vi "Untitled 1.vi"() -> ()   [LabVIEW 2021]
uses:
  <vilib>/Analysis/NI_AALPro.lvlib
panel:
  out "x*y":dbl
  out "x/y":dbl
  out "unsigned 16bit integer":u32 format="%x"
  out "output variable":dbl
  in  "Freq":dbl
  out "XY Graph":cluster{dbl[], dbl[]}(graph)
  out "intercept":dbl
  out "slope":dbl
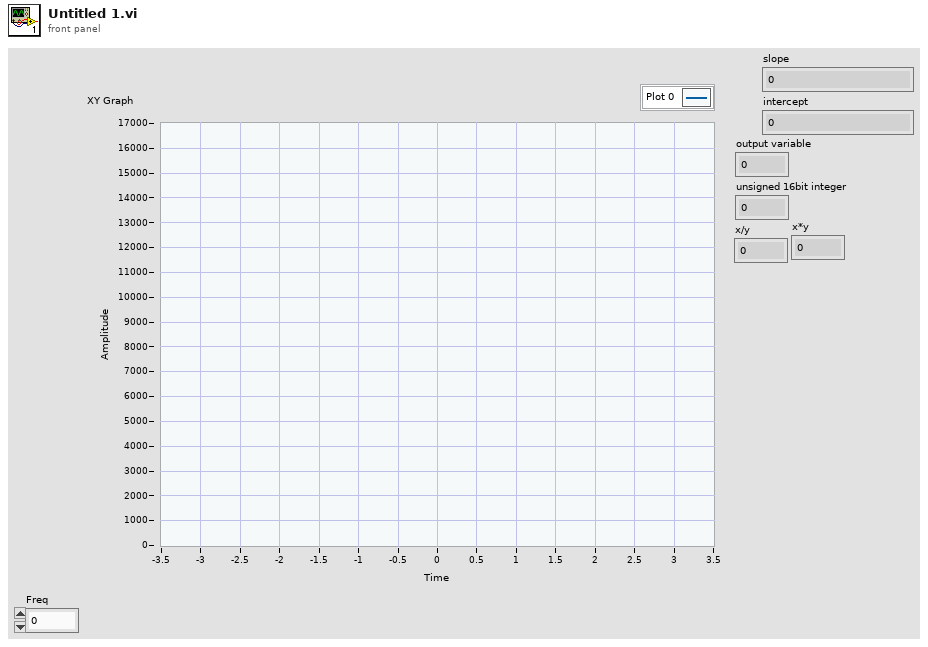
[diagram p1: front panel]
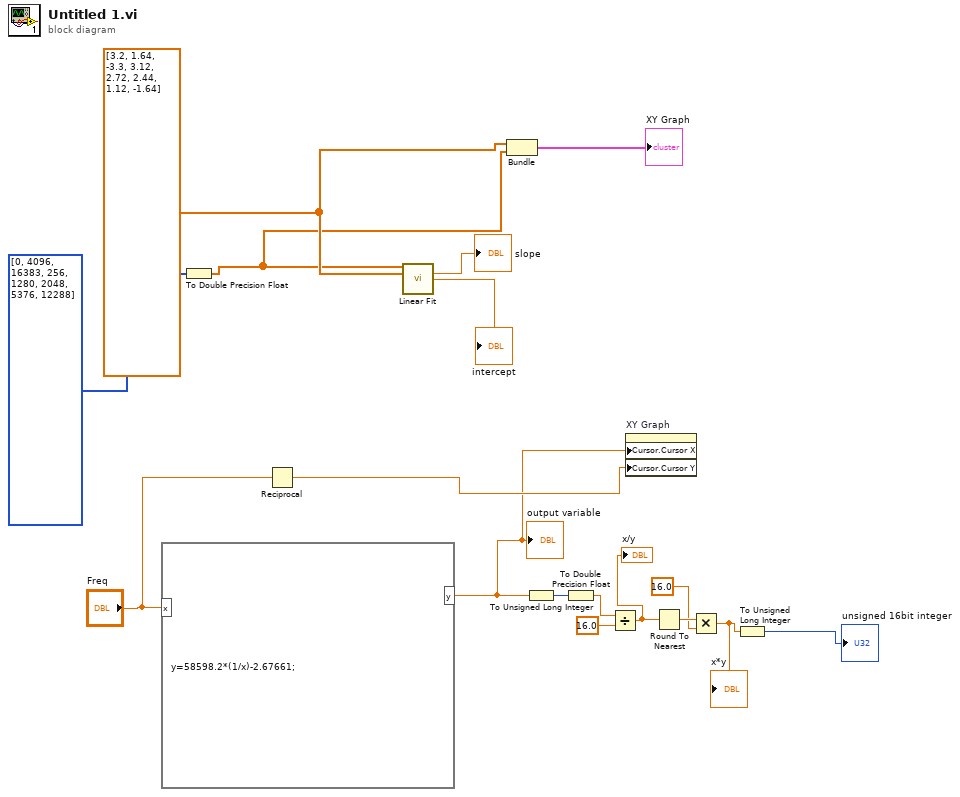
[diagram p0: block diagram]
diagram:
  w2 = dbl[] [3.2, 1.64, -3.3, 3.12, 2.72, 2.44, 1.12, -1.64]
  n1 = formula code="y=58598.2*(1/x)-2.67661;"("x"="Freq") -> ("y"=w11:dbl)
  "output variable" <- w11
  n2 = To Double Precision Float(number=i32[] [0, 4096, 16383, 256, 1280, 2048, 5376, 12288]) -> (double precision float=w1:dbl[])
  n3 = Reciprocal(x="Freq") -> (1/x=w12:dbl)
  n4 = call <vilib>:"Linear Fit.vi"("Y"=w1, "X"=w2) -> ("slope"=→"slope":dbl, "intercept"=→"intercept":dbl)  [unwired: 9 in, 3 out]
  n5 = Bundle(w2, w1) -> (→"XY Graph":cluster{dbl[], dbl[]})  [unwired: 1 in]
  n6 = To Unsigned Long Integer(number=w11) -> (unsigned 32bit integer=w10:u32)
  n7 = To Double Precision Float(number=w10) -> (double precision float=w9:dbl)
  n8 = Divide(x=w9, y=16.0) -> (x/y=w7:dbl)
  "x/y" <- w7
  n9 = property on="XY Graph" class="XYGraph (strict)"("Cursor.Cursor X"=w11, "Cursor.Cursor Y"=w12) -> ()  [unwired: 2 in, 2 out]
  n10 = Round To Nearest(number=w7) -> (nearest integer value=w6:dbl)
  n11 = Multiply(x=w6, y=16.0) -> (x*y=w4:dbl)
  "x*y" <- w4
  n12 = To Unsigned Long Integer(number=w4) -> (unsigned 32bit integer=→"unsigned 16bit integer":u32)
